vi "FileDialog.vi"(8 "error in":errorcluster, 11 "start path":path=path "") -> (0 "error out":errorcluster, 1 "cancelled":bool, 3 "selected path":path)   [LabVIEW 2013]
doc: "Opens a Dialog for getting the file Path for the configuration"
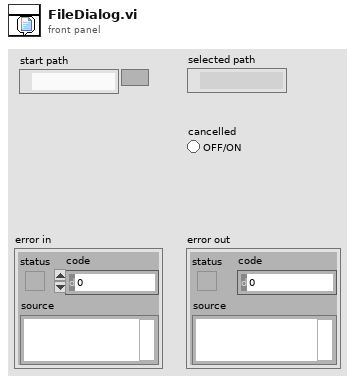
[diagram p1: front panel]
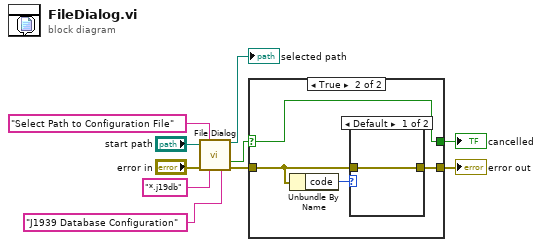
[diagram p0: block diagram]
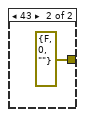
[diagram p3: hidden frame]
diagram:
  n1 = call "File Dialog"("start path"="start path", "prompt"="Select Path to Configuration File" ("Prompt"), "error in"="error in", "pattern (all files)"="*.j19db" ("pattern"), "pattern label"="J1939 Database Configuration") -> ("selected path"=→"selected path":path, "cancelled"=w9:bool, "error out"=w10:errorcluster)  [unwired: 7 in, 1 out]
  n2 = case shown="True" w9 {
    selector: w9 -> [w11 w13]
    tunnel: w10 -> [w12 w15]
    tunnel: [w12 w14] -> w7
    tunnel: [w11 w13] -> w8
    frame False {
    }
    frame True {
      n3 = Unbundle By Name(w15) -> ("code"=w16:i32)
      n4 = case shown="Default" w16 {
        tunnel: w15 -> [w17 _]
        tunnel: [w17 errorcluster {"status"=FALSE, "code"=0, "source"=""} ("error out")] -> w14
        frame Default {
        }
        frame 43 {
        }
      }
    }
  }
  "cancelled" <- w8
  "error out" <- w7
